vi "DaqOscilloscope2.vi"() -> ()   [LabVIEW 2025]
uses:
  <vilib>/DAQmx/read.llb/DAQmx Read (Analog 1D Wfm NChan NSamp).vi
  <vilib>/DAQmx/miscellaneous.llb/DAQmx Fill In Error Info.vi
panel:
  in  "stop":bool
  out "data":waveform(dbl)[](graph)
  out "error out":errorcluster
  in  "error in":errorcluster
  in  "physical channels":tag
  in  "channel settings":T1={"units"=10348, "input terminal configuration"=-1, "maximum value"=5.0, "minimum value"=-5.0} {"units" items=["Volts"=10348, "From Custom Scale"=10065]; "input terminal configuration" items=["Default"=-1, "RSE"=10083, "NRSE"=10078, "Differential"=10106, "Pseudodifferential"=12529]}
  in  "frequency settings":T2={"frequency (Hz)"=0.001, "number of samples per cycle"=2.0, "number of cycles"=1.0} {"frequency (Hz)" min=0.001 max=100000000.0; "number of samples per cycle" min=2.0 step=1.0; "number of cycles" min=1.0}
  # "Para usar la DAQ como osciloscopio"
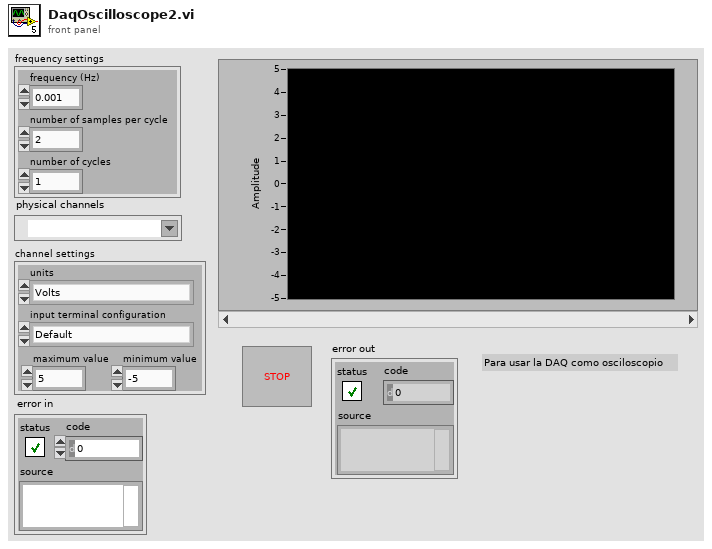
[diagram p1: front panel]
types:
  T1 = cluster{"units":i32, "input terminal configuration":i32, "maximum value":dbl, "minimum value":dbl}
  T2 = cluster{"frequency (Hz)":dbl, "number of samples per cycle":dbl, "number of cycles":dbl}
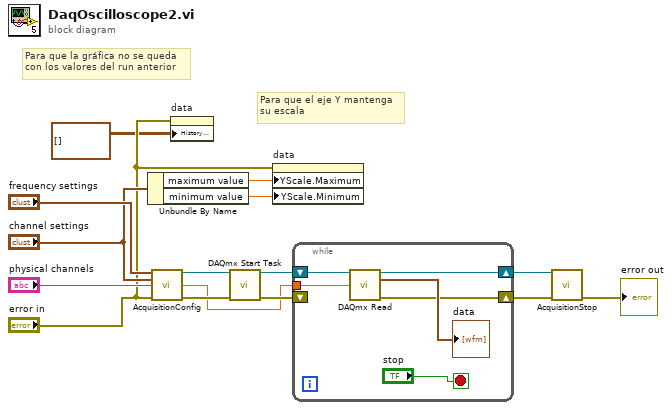
[diagram p0: block diagram]
diagram:
  # "Para que el eje Y mantenga\nsu escala"
  # "Para que la gráfica no se queda\ncon los valores del run anterior"
  n1 = Unbundle By Name("channel settings") -> ("maximum value"=w5:dbl, "minimum value"=w4:dbl)
  n2 = call "AcquisitionConfig.vi"("frequency settings"="frequency settings", "channel settings"="channel settings", "physical channels"="physical channels", "error in"="error in") -> ("task out"=w12:refnum<k21>, "number of samples"=w1:dbl, "error out"=w13:errorcluster)  [unwired: 9 in]
  n3 = property on="data" class="WFChart (strict)"(error in="error in", "History Data"=waveform(dbl)[][] []) -> ()  [unwired: 1 in, 2 out]
  n4 = call <vilib>:"DAQmx Start Task.vi"("task/channels in"=w12, "error in"=w13) -> ("task out"=w10:refnum<k21>, "error out"=w11:errorcluster)  [unwired: 12 in]
  n5 = property on="data" class="WFChart (strict)"(error in="error in", "YScale.Maximum"=w5, "YScale.Minimum"=w4) -> ()  [unwired: 1 in, 2 out]
  n6 = while {
    tunnel: w1 -> [w19]
    shift-right: [w16] -> w9
    shift-left: w11 -> [_]
    shift-right: [w20] -> w8
    shift-left: w10 -> [w21]
    stop <- "stop" stop-if-true
    n7 = call-poly <vilib>:"DAQmx Read.vi"("task/channels in"=w21, "number of samples per channel"=w19) -> ("task out"=w20:refnum<k21>, "data"=→"data":waveform(dbl)[], "error out"=w16:errorcluster)  [unwired: 11 in]
  }
  n8 = call "AcquisitionStop.vi"("task/channels in"=w8, "error in"=w9) -> ("error out"=→"error out":errorcluster)  [unwired: 13 in]
